vi "timekeeper clock.vi"   [LabVIEW 2011, in "EPS_Timekeeper.lvlib"]
uses:
  <vilib>/addons/Electrical Power/Example Support/PMU/Time Keeper/EPS_Timekeeper.lvlib
  <vilib>/Platform/TimedLoop/XDataNode/timing_clust.ctl
  <vilib>/Platform/TimedLoop/XDataNode/nitl_modes.ctl
  <vilib>/Platform/TimedLoop/XDataNode/wakeup.ctl
  <vilib>/rvi/FXPMathLib/FxpDiv/subVIs/nifxpmath_Div_SimConfig.ctl
  <vilib>/addons/Electrical Power/Example Support/PMU/Time Keeper/timekeeper time (g).vi
  <vilib>/addons/Electrical Power/Example Support/PMU/Time Keeper/timekeeper time rate adjust (g).vi
  <vilib>/addons/Electrical Power/Example Support/PMU/Time Keeper/timekeeper time rate adjust valid (g).vi
  <vilib>/addons/Electrical Power/Example Support/PMU/Time Keeper/timekeeper time adjustment update toggle (g).vi
  <vilib>/addons/Electrical Power/Example Support/PMU/Time Keeper/timekeeper time adjustment offset (g).vi
  <vilib>/rvi/FXPMathLib/FxpDiv/simVIs/DllFxpDivTemp_sub.vi
  <vilib>/Platform/TimedLoop/XDataNode/XDataNode.xnode
  <vilib>/rvi/FXPMathLib/FxpDiv/XNode/nifxpmath_Div.xnode
  <vilib>/Platform/TimedLoop/XDataNode/XDNodeRunTimeDep.lvlib
types:
  T1 = typedef "XDNodeRunTimeDep.lvlib/timing_clust.ctl" = cluster{"Expected End [f-1]":u64, "Actual End [f-1]":u64, "Finished Late? [f-1]":bool, "Expected End [i-1]":u64, "Actual End [i-1]":u64, "Finished Late? [i-1]":bool, "Expected Start [i]":u64, "Actual Start [i]":u64, "Expected Start [f]":u64, "Actual Start [f]":u64, "Source Name":string, "Structure Name":string, "Period":i64, "Deadline":i64, "Offset":i64, "Start":i64, "Priority":i32, "Timeout":i32, "Mode":T2, "Wakeup Reason":T3, "Error":errorcluster, "Source Type":string, "Secondary Source Type":string, "Global End Time":u64, "Global Start Time":u64, "Frame Duration":u64, "Iteration Duration":u64, "Assigned CPU":i32, "I/O Scan Engine Mode":u32}
  T2 = typedef "XDNodeRunTimeDep.lvlib/nitl_modes.ctl" = enum32{"No Change", "Process missed periods, maintain original phase", "Discard missed periods, maintain original phase", "Process missed periods, ignore original phase", "Discard missed periods, ignore original phase"}
  T3 = typedef "XDNodeRunTimeDep.lvlib/wakeup.ctl" = enum32{"Normal", "Aborted", "Asynchronous wakeup", "Timing source error", "Timed loop error", "Timeout"}
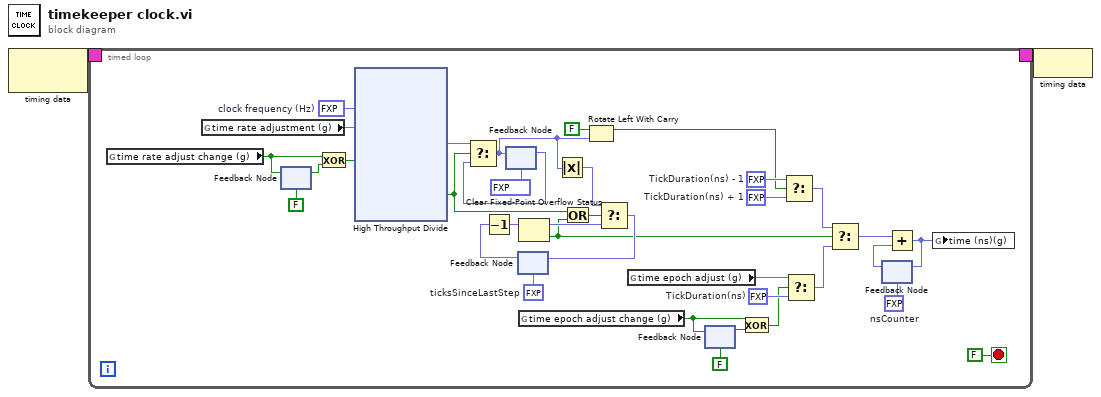
[diagram p0: block diagram]
diagram:
  n1 = node-c288() -> (w2:T1)  [unwired: 1 in]
  n2 = timed-loop "Timed Loop" {
    timing: w2 -> [_]
    timing-out: [_] -> w1
    stop <- FALSE stop-if-true
    w25 = fxp<+,5,5> 26.0  # TickDuration(ns) + 1
    w26 = fxp<+,5,5> 24.0  # TickDuration(ns) - 1
    w16 = fxp<+,5,5> 25.0  # TickDuration(ns)
    w28 = fxp<+,26,26> 40000000.0  # clock frequency (Hz)
    w32 = fxp<+,26,26> 0.0  # ticksSinceLastStep
    w35 = fxp<+,64,64> 0.0  # nsCounter
    n3 = global read "timekeeper time rate adjust valid (g).vi" "time rate adjust change (g)"() -> (w21:bool)
    n4 = global read "timekeeper time rate adjust (g).vi" "time rate adjustment (g)"() -> (w4:fxp<+/-,19,19>)
    n5 = feedback #1(FALSE ("input valid")) -> (w20:bool)
    n6 = feedback-in #1(w21) -> ()
    n7 = Exclusive Or(1:w20, 2:w21) -> (0:w27:bool)
    n8 = xnode "High Throughput Divide"("x"=w28, "y"=w4, "input valid"=w27) -> ("x/y"=w11:fxp<+/-,27,27>, "output valid"=w7:bool)  [unwired: 1 in, 1 out]
    n9 = feedback #2(fxp<+/-,27,27> 40000000.0 ("x/y")) -> (w10:fxp<+/-,27,27>)
    n10 = Select(t=w11, s=w7, f=w10) -> (s? t:f=w5:fxp<+/-,27,27>)
    n11 = feedback-in #2(w5) -> ()
    n12 = feedback #3(w32) -> (w31:fxp<+,27,27>)
    n13 = Decrement(x=w31) -> (x-1=w37:fxp<+,26,26>)
    n14 = Clear Fixed-Point Overflow Status(3:w37) -> (0:w6:bool, 1:w30:fxp<+,26,26>)
    n15 = global read "timekeeper time adjustment update toggle (g).vi" "time epoch adjust change (g)"() -> (w17:bool)
    n16 = Absolute Value(x=w5) -> (abs(x)=w9:fxp<+,27,27>)
    n17 = Or(x=w7, y=w6) -> (x .or. y?=w8:bool)
    n18 = Rotate Left With Carry(2:w5, 3:FALSE ("carry")) -> (1:w23:bool)  [unwired: 1 out]
    n19 = Select(t=w9, s=w8, f=w30) -> (s? t:f=w29:fxp<+,27,27>)
    n20 = feedback-in #3(w29) -> ()
    n21 = global read "timekeeper time adjustment offset (g).vi" "time epoch adjust (g)"() -> (w15:fxp<+/-,64,64>)
    n22 = feedback #4(FALSE ("input valid")) -> (w18:bool)
    n23 = feedback-in #4(w17) -> ()
    n24 = Exclusive Or(1:w18, 2:w17) -> (0:w14:bool)
    n25 = Select(t=w26, s=w23, f=w25) -> (s? t:f=w24:fxp<+,5,5>)
    n26 = Select(t=w15, s=w14, f=w16) -> (s? t:f=w13:fxp<+/-,64,64>)
    n27 = Select(t=w24, s=w6, f=w13) -> (s? t:f=w22:fxp<+/-,64,64>)
    n28 = feedback #5(w35) -> (w34:fxp<+,64,64>)
    n29 = Add(x=w22, y=w34) -> (x+y=w3:fxp<+,64,64>)
    n30 = feedback-in #5(w3) -> ()
    n31 = global write "timekeeper time (g).vi" "time (ns)(g)"(w3) -> ()
  }
  n32 = node-c288(w1) -> ()
